vi "Pack Bits x8 (SubVI).vi"(0 "Input Valid?":bool, 2 "Data In":T1, 5 "Bit Depth":u8) -> (14 "Output Valid?":bool, 16 "Data Out":u8[](array[numeric]), 18 "Pixel Sync":bool, 19 "N Bytes":u8)   [LabVIEW 2015]
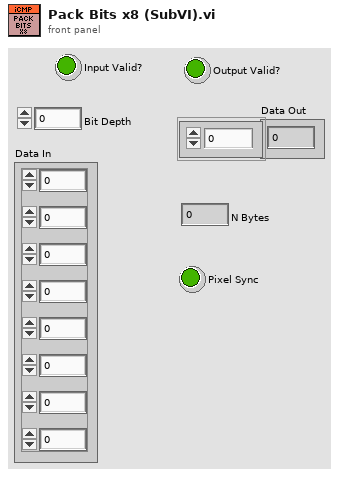
[diagram p1: front panel]
types:
  T1 = cluster{"Numeric Control":u8, "Numeric Control":u8, "Numeric Control":u8, "Numeric Control":u8, "Numeric Control":u8, "Numeric Control":u8, "Numeric Control":u8, "Numeric Control":u8}
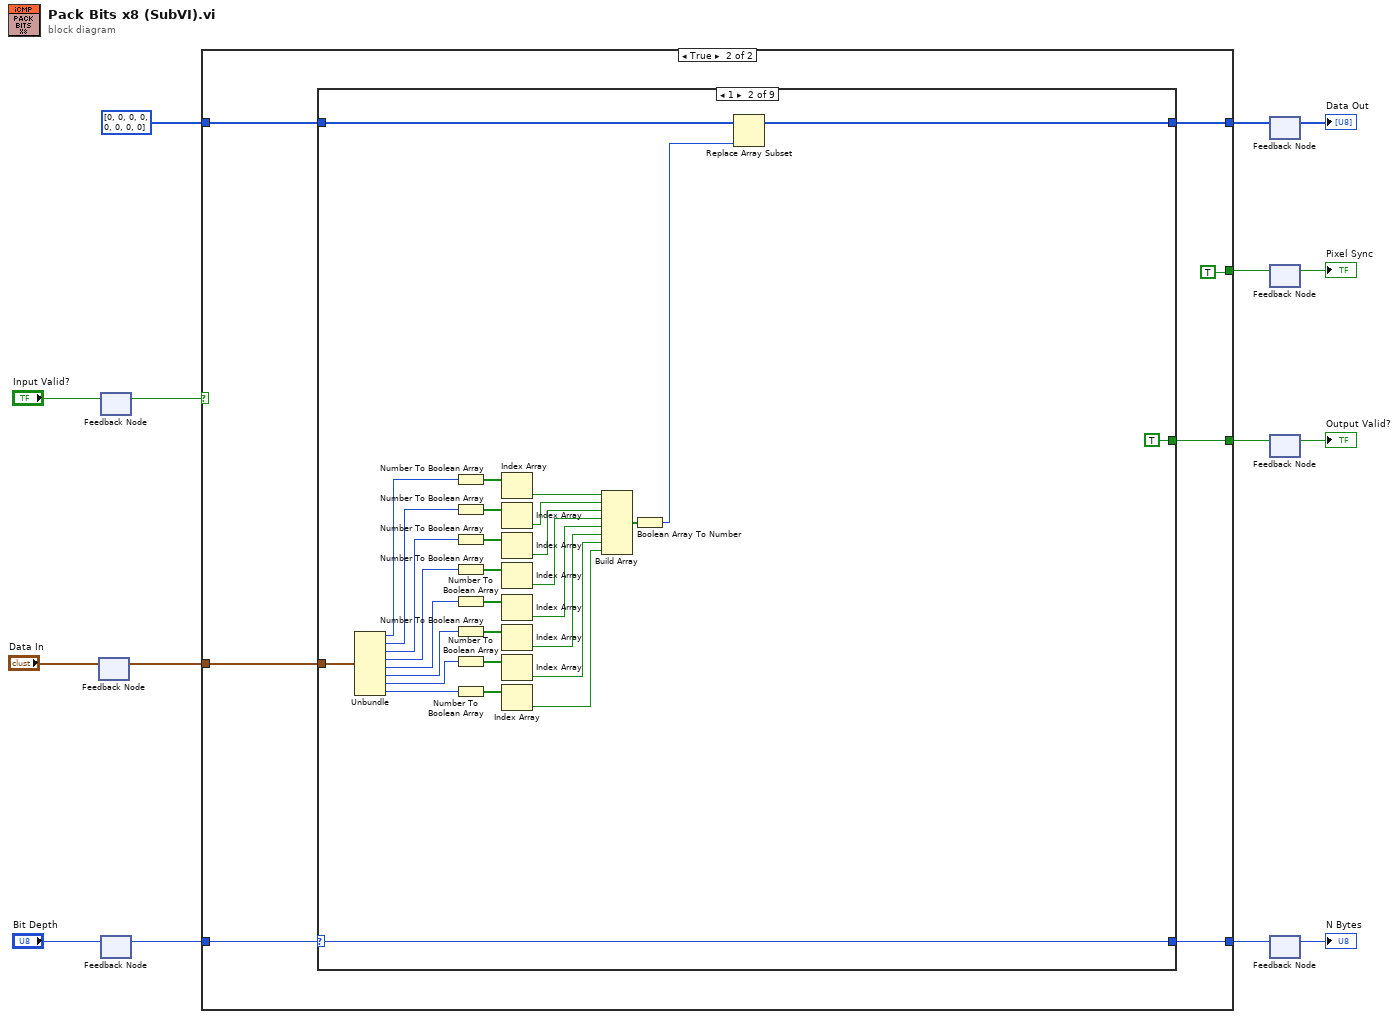
[diagram p0: block diagram]
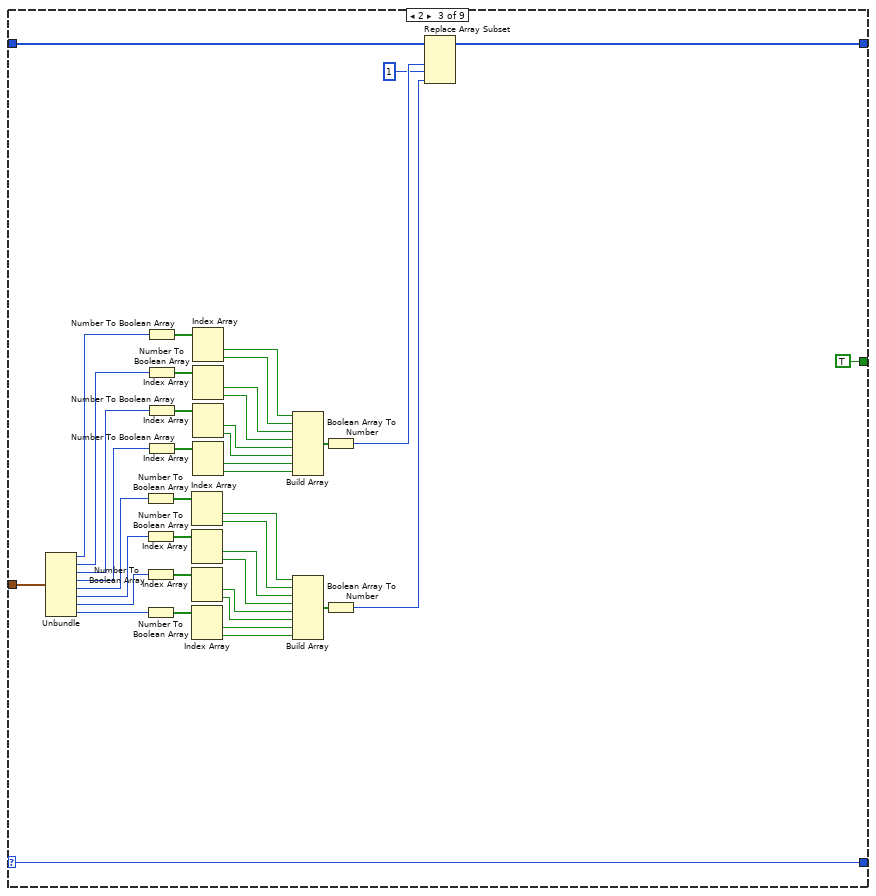
[diagram p4: hidden frame]
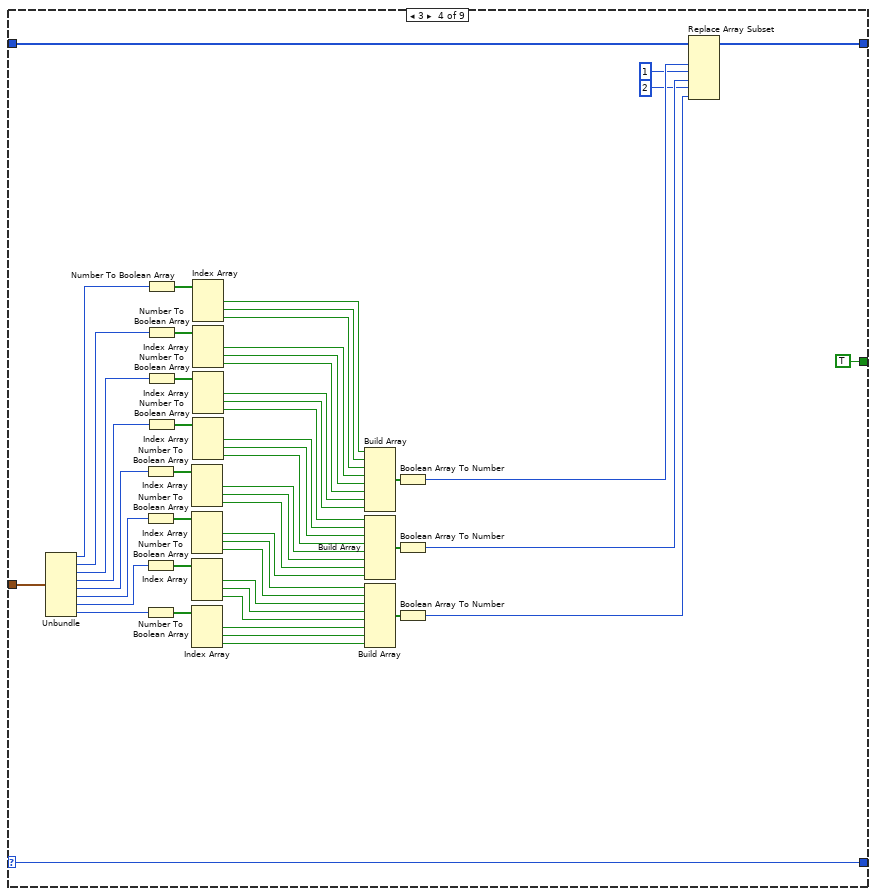
[diagram p5: hidden frame]
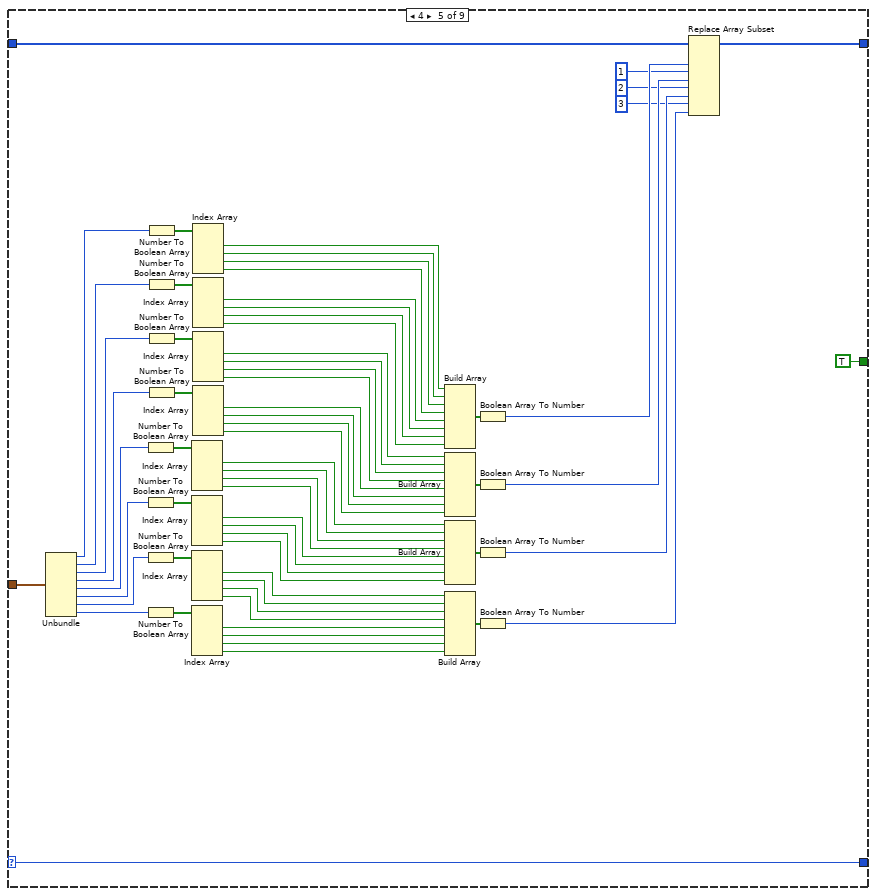
[diagram p6: hidden frame]
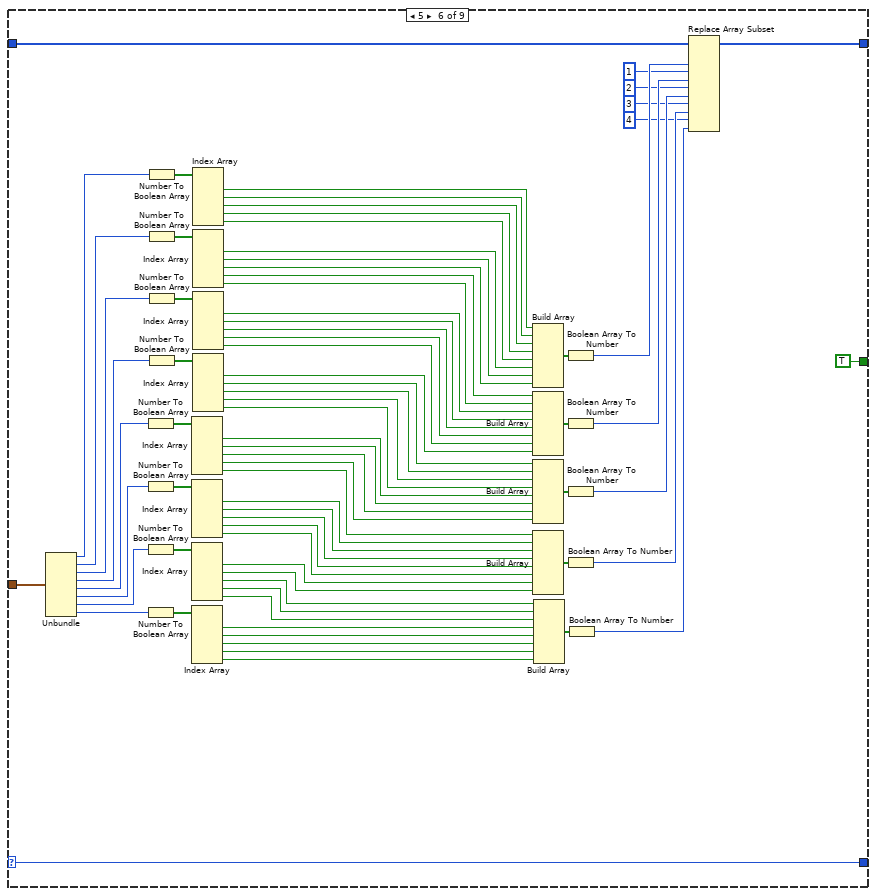
[diagram p7: hidden frame]
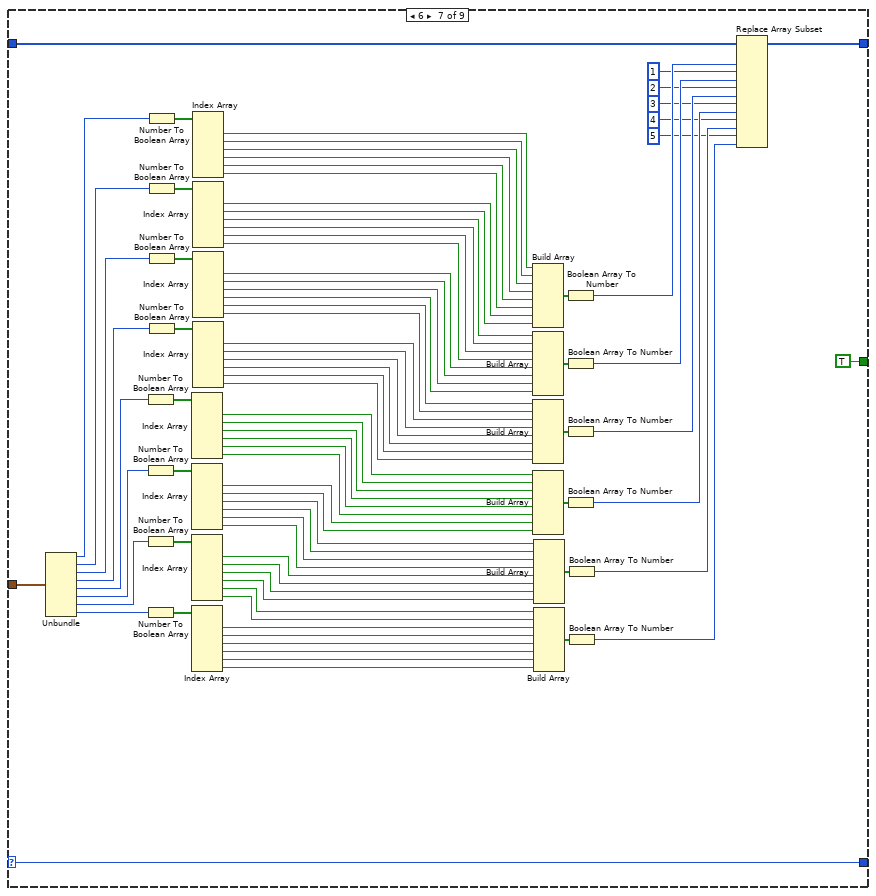
[diagram p8: hidden frame]
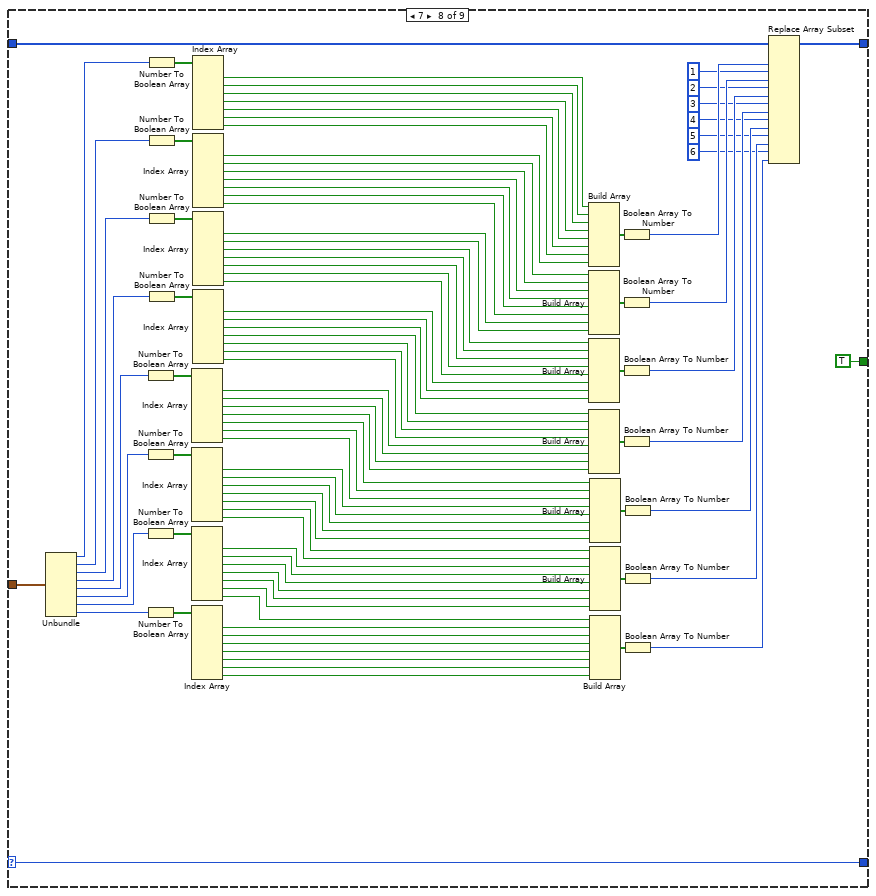
[diagram p9: hidden frame]
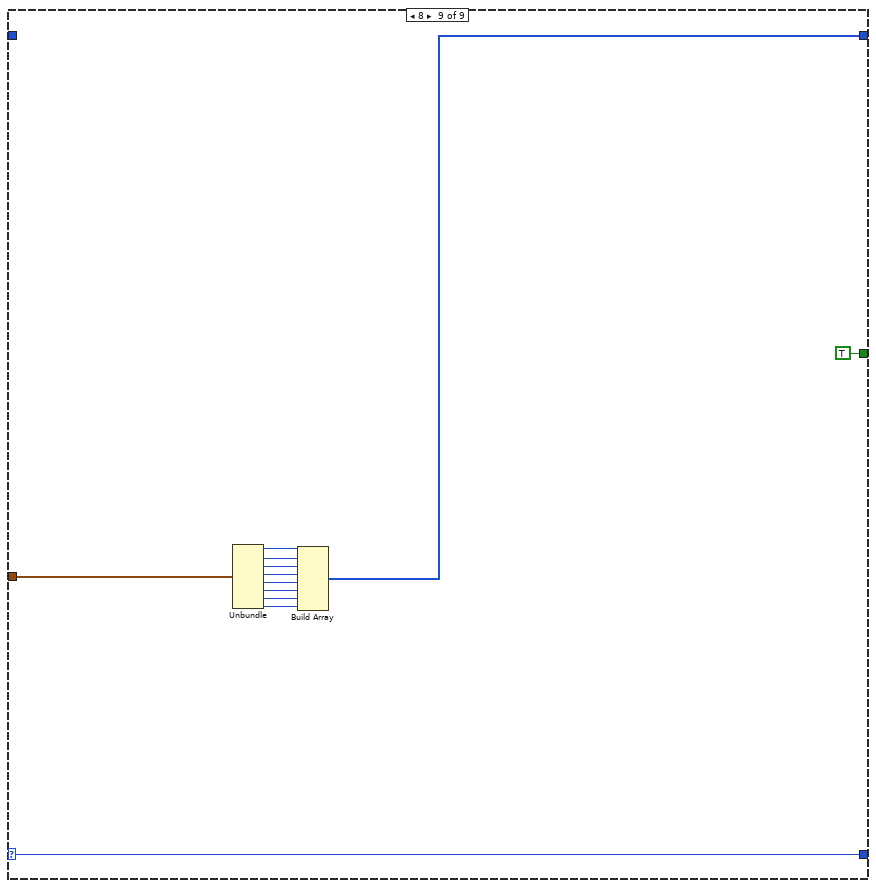
[diagram p10: hidden frame]
diagram:
  n1 = feedback-in #1("Data In") -> ()
  n2 = feedback #1() -> (w11:T1)  [unwired: 1 in]
  n3 = feedback-in #2("Input Valid?") -> ()
  n4 = feedback #2() -> (w13:bool)  [unwired: 1 in]
  n5 = feedback-in #3("Bit Depth") -> ()
  n6 = feedback #3() -> (w10:u8)  [unwired: 1 in]
  n7 = case shown="True" w13 {
    tunnel: [_ w20] -> w8
    tunnel: w11 -> [_ w18]
    tunnel: w10 -> [_ w23]
    tunnel: u8[] [0, 0, 0, 0, 0, 0, 0, 0] -> [w16 w22]
    tunnel: [w16 w21] -> w6
    tunnel: [_ w19] -> w7
    tunnel: [_ TRUE] -> w1
    frame False {
    }
    frame True {
      n8 = case shown="1" w23 {
        selector: w23 -> [w25 w27 w58 w129 w193 w268 w354 w451 w485]
        tunnel: w18 -> [_ w56 w98 w151 w215 w290 w376 w473 w476]
        tunnel: w22 -> [w24 w30 w88 w142 w206 w281 w367 w464 _]
        tunnel: [w24 w28 w86 w140 w204 w279 w365 w462 w475] -> w21
        tunnel: [_ TRUE TRUE TRUE TRUE TRUE TRUE TRUE TRUE] -> w20
        tunnel: [w25 w27 w58 w129 w193 w268 w354 w451 w485] -> w19
        frame 0, Default {
        }
        frame 1 {
          n9 = Unbundle(w56) -> ("Numeric Control"=w55:u8, "Numeric Control"=w52:u8, "Numeric Control"=w49:u8, "Numeric Control"=w48:u8, "Numeric Control"=w43:u8, "Numeric Control"=w42:u8, "Numeric Control"=w41:u8, "Numeric Control"=w40:u8)
          n10 = Number To Boolean Array(number=w55) -> (Boolean array=w54:bool[])
          n11 = Number To Boolean Array(number=w52) -> (Boolean array=w53:bool[])
          n12 = Number To Boolean Array(number=w49) -> (Boolean array=w50:bool[])
          n13 = Number To Boolean Array(number=w48) -> (Boolean array=w51:bool[])
          n14 = Number To Boolean Array(number=w43) -> (Boolean array=w44:bool[])
          n15 = Number To Boolean Array(number=w42) -> (Boolean array=w45:bool[])
          n16 = Number To Boolean Array(number=w41) -> (Boolean array=w47:bool[])
          n17 = Number To Boolean Array(number=w40) -> (Boolean array=w46:bool[])
          n18 = Index Array(array=w54) -> (element=w39:bool)  [unwired: 1 in]
          n19 = Index Array(array=w53) -> (element=w38:bool)  [unwired: 1 in]
          n20 = Index Array(array=w50) -> (element=w37:bool)  [unwired: 1 in]
          n21 = Index Array(array=w51) -> (element=w36:bool)  [unwired: 1 in]
          n22 = Index Array(array=w44) -> (element=w35:bool)  [unwired: 1 in]
          n23 = Index Array(array=w45) -> (element=w34:bool)  [unwired: 1 in]
          n24 = Index Array(array=w47) -> (element=w33:bool)  [unwired: 1 in]
          n25 = Index Array(array=w46) -> (element=w32:bool)  [unwired: 1 in]
          n26 = Build Array(w39, w38, w37, w36, w35, w34, w33, w32) -> (w31:bool[])
          n27 = Boolean Array To Number(Boolean array=w31) -> (number=w29:u8)
          n28 = Replace Array Subset(array=w30, new element=w29) -> (w28:u8[])  [unwired: 1 in]
        }
        frame 2 {
          n29 = Unbundle(w98) -> ("Numeric Control"=w97:u8, "Numeric Control"=w94:u8, "Numeric Control"=w91:u8, "Numeric Control"=w90:u8, "Numeric Control"=w62:u8, "Numeric Control"=w61:u8, "Numeric Control"=w60:u8, "Numeric Control"=w59:u8)
          n30 = Number To Boolean Array(number=w62) -> (Boolean array=w64:bool[])
          n31 = Number To Boolean Array(number=w61) -> (Boolean array=w65:bool[])
          n32 = Number To Boolean Array(number=w60) -> (Boolean array=w67:bool[])
          n33 = Number To Boolean Array(number=w59) -> (Boolean array=w66:bool[])
          n34 = Number To Boolean Array(number=w97) -> (Boolean array=w96:bool[])
          n35 = Number To Boolean Array(number=w94) -> (Boolean array=w95:bool[])
          n36 = Number To Boolean Array(number=w91) -> (Boolean array=w92:bool[])
          n37 = Number To Boolean Array(number=w90) -> (Boolean array=w93:bool[])
          n38 = Index Array(array=w64) -> (element #1=w69:bool, element #2=w70:bool)  [unwired: 2 in]
          n39 = Index Array(array=w65) -> (element #1=w71:bool, element #2=w72:bool)  [unwired: 2 in]
          n40 = Index Array(array=w67) -> (element #1=w73:bool, element #2=w74:bool)  [unwired: 2 in]
          n41 = Index Array(array=w66) -> (element #1=w75:bool, element #2=w76:bool)  [unwired: 2 in]
          n42 = Index Array(array=w96) -> (element #1=w84:bool, element #2=w83:bool)  [unwired: 2 in]
          n43 = Index Array(array=w95) -> (element #1=w82:bool, element #2=w81:bool)  [unwired: 2 in]
          n44 = Index Array(array=w92) -> (element #1=w80:bool, element #2=w79:bool)  [unwired: 2 in]
          n45 = Index Array(array=w93) -> (element #1=w78:bool, element #2=w77:bool)  [unwired: 2 in]
          n46 = Build Array(w84, w83, w82, w81, w80, w79, w78, w77) -> (w89:bool[])
          n47 = Build Array(w69, w70, w71, w72, w73, w74, w75, w76) -> (w68:bool[])
          n48 = Boolean Array To Number(Boolean array=w89) -> (number=w87:u8)
          n49 = Boolean Array To Number(Boolean array=w68) -> (number=w63:u8)
          n50 = Replace Array Subset(array=w88, new element #1=w87, new element #2=w63, index #2=1 ("index")) -> (w86:u8[])  [unwired: 1 in]
        }
        frame 3 {
          n51 = Unbundle(w151) -> ("Numeric Control"=w150:u8, "Numeric Control"=w147:u8, "Numeric Control"=w144:u8, "Numeric Control"=w143:u8, "Numeric Control"=w133:u8, "Numeric Control"=w132:u8, "Numeric Control"=w131:u8, "Numeric Control"=w130:u8)
          n52 = Number To Boolean Array(number=w133) -> (Boolean array=w135:bool[])
          n53 = Number To Boolean Array(number=w132) -> (Boolean array=w136:bool[])
          n54 = Number To Boolean Array(number=w131) -> (Boolean array=w138:bool[])
          n55 = Number To Boolean Array(number=w130) -> (Boolean array=w137:bool[])
          n56 = Number To Boolean Array(number=w150) -> (Boolean array=w149:bool[])
          n57 = Number To Boolean Array(number=w147) -> (Boolean array=w148:bool[])
          n58 = Number To Boolean Array(number=w144) -> (Boolean array=w145:bool[])
          n59 = Number To Boolean Array(number=w143) -> (Boolean array=w146:bool[])
          n60 = Index Array(array=w135) -> (element #1=w114:bool, element #2=w113:bool, element #3=w112:bool)  [unwired: 3 in]
          n61 = Index Array(array=w136) -> (element #1=w111:bool, element #2=w107:bool, element #3=w106:bool)  [unwired: 3 in]
          n62 = Index Array(array=w138) -> (element #1=w105:bool, element #2=w104:bool, element #3=w103:bool)  [unwired: 3 in]
          n63 = Index Array(array=w137) -> (element #1=w102:bool, element #2=w101:bool, element #3=w100:bool)  [unwired: 3 in]
          n64 = Index Array(array=w149) -> (element #1=w126:bool, element #2=w125:bool, element #3=w124:bool)  [unwired: 3 in]
          n65 = Index Array(array=w148) -> (element #1=w123:bool, element #2=w122:bool, element #3=w121:bool)  [unwired: 3 in]
          n66 = Index Array(array=w145) -> (element #1=w120:bool, element #2=w119:bool, element #3=w118:bool)  [unwired: 3 in]
          n67 = Index Array(array=w146) -> (element #1=w117:bool, element #2=w116:bool, element #3=w115:bool)  [unwired: 3 in]
          n68 = Build Array(w126, w125, w124, w123, w122, w121, w120, w119) -> (w128:bool[])
          n69 = Build Array(w118, w117, w116, w115, w114, w113, w112, w111) -> (w127:bool[])
          n70 = Build Array(w107, w106, w105, w104, w103, w102, w101, w100) -> (w109:bool[])
          n71 = Boolean Array To Number(Boolean array=w128) -> (number=w141:u8)
          n72 = Boolean Array To Number(Boolean array=w127) -> (number=w134:u8)
          n73 = Boolean Array To Number(Boolean array=w109) -> (number=w108:u8)
          n74 = Replace Array Subset(array=w142, new element #1=w141, new element #2=w134, index #2=1 ("index"), new element #3=w108, index #3=2 ("index")) -> (w140:u8[])  [unwired: 1 in]
        }
        frame 4 {
          n75 = Unbundle(w215) -> ("Numeric Control"=w214:u8, "Numeric Control"=w211:u8, "Numeric Control"=w208:u8, "Numeric Control"=w207:u8, "Numeric Control"=w197:u8, "Numeric Control"=w196:u8, "Numeric Control"=w195:u8, "Numeric Control"=w194:u8)
          n76 = Number To Boolean Array(number=w197) -> (Boolean array=w199:bool[])
          n77 = Number To Boolean Array(number=w196) -> (Boolean array=w200:bool[])
          n78 = Number To Boolean Array(number=w195) -> (Boolean array=w202:bool[])
          n79 = Number To Boolean Array(number=w194) -> (Boolean array=w201:bool[])
          n80 = Number To Boolean Array(number=w214) -> (Boolean array=w213:bool[])
          n81 = Number To Boolean Array(number=w211) -> (Boolean array=w212:bool[])
          n82 = Number To Boolean Array(number=w208) -> (Boolean array=w209:bool[])
          n83 = Number To Boolean Array(number=w207) -> (Boolean array=w210:bool[])
          n84 = Index Array(array=w199) -> (element #1=w168:bool, element #2=w167:bool, element #3=w166:bool, element #4=w165:bool)  [unwired: 4 in]
          n85 = Index Array(array=w200) -> (element #1=w164:bool, element #2=w163:bool, element #3=w162:bool, element #4=w161:bool)  [unwired: 4 in]
          n86 = Index Array(array=w202) -> (element #1=w160:bool, element #2=w159:bool, element #3=w158:bool, element #4=w157:bool)  [unwired: 4 in]
          n87 = Index Array(array=w201) -> (element #1=w156:bool, element #2=w155:bool, element #3=w154:bool, element #4=w153:bool)  [unwired: 4 in]
          n88 = Index Array(array=w213) -> (element #1=w190:bool, element #2=w189:bool, element #3=w188:bool, element #4=w181:bool)  [unwired: 4 in]
          n89 = Index Array(array=w212) -> (element #1=w180:bool, element #2=w179:bool, element #3=w178:bool, element #4=w177:bool)  [unwired: 4 in]
          n90 = Index Array(array=w209) -> (element #1=w176:bool, element #2=w175:bool, element #3=w174:bool, element #4=w173:bool)  [unwired: 4 in]
          n91 = Index Array(array=w210) -> (element #1=w172:bool, element #2=w171:bool, element #3=w170:bool, element #4=w169:bool)  [unwired: 4 in]
          n92 = Build Array(w190, w189, w188, w181, w180, w179, w178, w177) -> (w192:bool[])
          n93 = Build Array(w176, w175, w174, w173, w172, w171, w170, w169) -> (w191:bool[])
          n94 = Build Array(w168, w167, w166, w165, w164, w163, w162, w161) -> (w186:bool[])
          n95 = Build Array(w160, w159, w158, w157, w156, w155, w154, w153) -> (w184:bool[])
          n96 = Boolean Array To Number(Boolean array=w192) -> (number=w205:u8)
          n97 = Boolean Array To Number(Boolean array=w191) -> (number=w198:u8)
          n98 = Boolean Array To Number(Boolean array=w186) -> (number=w185:u8)
          n99 = Boolean Array To Number(Boolean array=w184) -> (number=w182:u8)
          n100 = Replace Array Subset(array=w206, new element #1=w205, new element #2=w198, index #2=1 ("index"), new element #3=w185, index #3=2 ("index"), new element #4=w182, index #4=3 ("index")) -> (w204:u8[])  [unwired: 1 in]
        }
        frame 5 {
          n101 = Unbundle(w290) -> ("Numeric Control"=w289:u8, "Numeric Control"=w286:u8, "Numeric Control"=w283:u8, "Numeric Control"=w282:u8, "Numeric Control"=w272:u8, "Numeric Control"=w271:u8, "Numeric Control"=w270:u8, "Numeric Control"=w269:u8)
          n102 = Number To Boolean Array(number=w272) -> (Boolean array=w274:bool[])
          n103 = Number To Boolean Array(number=w271) -> (Boolean array=w275:bool[])
          n104 = Number To Boolean Array(number=w270) -> (Boolean array=w277:bool[])
          n105 = Number To Boolean Array(number=w269) -> (Boolean array=w276:bool[])
          n106 = Number To Boolean Array(number=w289) -> (Boolean array=w288:bool[])
          n107 = Number To Boolean Array(number=w286) -> (Boolean array=w287:bool[])
          n108 = Number To Boolean Array(number=w283) -> (Boolean array=w284:bool[])
          n109 = Number To Boolean Array(number=w282) -> (Boolean array=w285:bool[])
          n110 = Index Array(array=w274) -> (element #1=w236:bool, element #2=w235:bool, element #3=w234:bool, element #4=w233:bool, element #5=w232:bool)  [unwired: 5 in]
          n111 = Index Array(array=w275) -> (element #1=w231:bool, element #2=w230:bool, element #3=w229:bool, element #4=w228:bool, element #5=w227:bool)  [unwired: 5 in]
          n112 = Index Array(array=w277) -> (element #1=w226:bool, element #2=w225:bool, element #3=w224:bool, element #4=w223:bool, element #5=w222:bool)  [unwired: 5 in]
          n113 = Index Array(array=w276) -> (element #1=w221:bool, element #2=w220:bool, element #3=w219:bool, element #4=w218:bool, element #5=w217:bool)  [unwired: 5 in]
          n114 = Index Array(array=w288) -> (element #1=w265:bool, element #2=w264:bool, element #3=w263:bool, element #4=w256:bool, element #5=w252:bool)  [unwired: 5 in]
          n115 = Index Array(array=w287) -> (element #1=w251:bool, element #2=w250:bool, element #3=w249:bool, element #4=w248:bool, element #5=w247:bool)  [unwired: 5 in]
          n116 = Index Array(array=w284) -> (element #1=w246:bool, element #2=w245:bool, element #3=w244:bool, element #4=w243:bool, element #5=w242:bool)  [unwired: 5 in]
          n117 = Index Array(array=w285) -> (element #1=w241:bool, element #2=w240:bool, element #3=w239:bool, element #4=w238:bool, element #5=w237:bool)  [unwired: 5 in]
          n118 = Build Array(w265, w264, w263, w256, w252, w251, w250, w249) -> (w267:bool[])
          n119 = Build Array(w248, w247, w246, w245, w244, w243, w242, w241) -> (w266:bool[])
          n120 = Build Array(w240, w239, w238, w237, w236, w235, w234, w233) -> (w261:bool[])
          n121 = Build Array(w232, w231, w230, w229, w228, w227, w226, w225) -> (w259:bool[])
          n122 = Build Array(w224, w223, w222, w221, w220, w219, w218, w217) -> (w255:bool[])
          n123 = Boolean Array To Number(Boolean array=w267) -> (number=w280:u8)
          n124 = Boolean Array To Number(Boolean array=w266) -> (number=w273:u8)
          n125 = Boolean Array To Number(Boolean array=w261) -> (number=w260:u8)
          n126 = Boolean Array To Number(Boolean array=w259) -> (number=w257:u8)
          n127 = Boolean Array To Number(Boolean array=w255) -> (number=w253:u8)
          n128 = Replace Array Subset(array=w281, new element #1=w280, new element #2=w273, index #2=1 ("index"), new element #3=w260, index #3=2 ("index"), new element #4=w257, index #4=3 ("index"), new element #5=w253, index #5=4 ("index")) -> (w279:u8[])  [unwired: 1 in]
        }
        frame 6 {
          n129 = Unbundle(w376) -> ("Numeric Control"=w375:u8, "Numeric Control"=w372:u8, "Numeric Control"=w369:u8, "Numeric Control"=w368:u8, "Numeric Control"=w358:u8, "Numeric Control"=w357:u8, "Numeric Control"=w356:u8, "Numeric Control"=w355:u8)
          n130 = Number To Boolean Array(number=w358) -> (Boolean array=w360:bool[])
          n131 = Number To Boolean Array(number=w357) -> (Boolean array=w361:bool[])
          n132 = Number To Boolean Array(number=w356) -> (Boolean array=w363:bool[])
          n133 = Number To Boolean Array(number=w355) -> (Boolean array=w362:bool[])
          n134 = Number To Boolean Array(number=w375) -> (Boolean array=w374:bool[])
          n135 = Number To Boolean Array(number=w372) -> (Boolean array=w373:bool[])
          n136 = Number To Boolean Array(number=w369) -> (Boolean array=w370:bool[])
          n137 = Number To Boolean Array(number=w368) -> (Boolean array=w371:bool[])
          n138 = Index Array(array=w360) -> (element #1=w315:bool, element #2=w314:bool, element #3=w313:bool, element #4=w312:bool, element #5=w311:bool, element #6=w310:bool)  [unwired: 6 in]
          n139 = Index Array(array=w361) -> (element #1=w309:bool, element #2=w308:bool, element #3=w307:bool, element #4=w306:bool, element #5=w305:bool, element #6=w304:bool)  [unwired: 6 in]
          n140 = Index Array(array=w363) -> (element #1=w303:bool, element #2=w302:bool, element #3=w301:bool, element #4=w300:bool, element #5=w299:bool, element #6=w298:bool)  [unwired: 6 in]
          n141 = Index Array(array=w362) -> (element #1=w297:bool, element #2=w296:bool, element #3=w295:bool, element #4=w294:bool, element #5=w293:bool, element #6=w292:bool)  [unwired: 6 in]
          n142 = Index Array(array=w374) -> (element #1=w351:bool, element #2=w350:bool, element #3=w349:bool, element #4=w342:bool, element #5=w338:bool, element #6=w334:bool)  [unwired: 6 in]
          n143 = Index Array(array=w373) -> (element #1=w333:bool, element #2=w332:bool, element #3=w331:bool, element #4=w330:bool, element #5=w329:bool, element #6=w328:bool)  [unwired: 6 in]
          n144 = Index Array(array=w370) -> (element #1=w327:bool, element #2=w326:bool, element #3=w325:bool, element #4=w324:bool, element #5=w323:bool, element #6=w322:bool)  [unwired: 6 in]
          n145 = Index Array(array=w371) -> (element #1=w321:bool, element #2=w320:bool, element #3=w319:bool, element #4=w318:bool, element #5=w317:bool, element #6=w316:bool)  [unwired: 6 in]
          n146 = Build Array(w351, w350, w349, w342, w338, w334, w333, w332) -> (w353:bool[])
          n147 = Build Array(w331, w330, w329, w328, w327, w326, w325, w324) -> (w352:bool[])
          n148 = Build Array(w323, w322, w321, w320, w319, w318, w317, w316) -> (w347:bool[])
          n149 = Build Array(w315, w314, w313, w312, w311, w310, w309, w308) -> (w345:bool[])
          n150 = Build Array(w307, w306, w305, w304, w303, w302, w301, w300) -> (w341:bool[])
          n151 = Build Array(w299, w298, w297, w296, w295, w294, w293, w292) -> (w336:bool[])
          n152 = Boolean Array To Number(Boolean array=w353) -> (number=w366:u8)
          n153 = Boolean Array To Number(Boolean array=w352) -> (number=w359:u8)
          n154 = Boolean Array To Number(Boolean array=w347) -> (number=w346:u8)
          n155 = Boolean Array To Number(Boolean array=w345) -> (number=w343:u8)
          n156 = Boolean Array To Number(Boolean array=w341) -> (number=w339:u8)
          n157 = Boolean Array To Number(Boolean array=w336) -> (number=w335:u8)
          n158 = Replace Array Subset(array=w367, new element #1=w366, new element #2=w359, index #2=1 ("index"), new element #3=w346, index #3=2 ("index"), new element #4=w343, index #4=3 ("index"), new element #5=w339, index #5=4 ("index"), new element #6=w335, index #6=5 ("index")) -> (w365:u8[])  [unwired: 1 in]
        }
        frame 7 {
          n159 = Unbundle(w473) -> ("Numeric Control"=w472:u8, "Numeric Control"=w469:u8, "Numeric Control"=w466:u8, "Numeric Control"=w465:u8, "Numeric Control"=w455:u8, "Numeric Control"=w454:u8, "Numeric Control"=w453:u8, "Numeric Control"=w452:u8)
          n160 = Number To Boolean Array(number=w455) -> (Boolean array=w457:bool[])
          n161 = Number To Boolean Array(number=w454) -> (Boolean array=w458:bool[])
          n162 = Number To Boolean Array(number=w453) -> (Boolean array=w460:bool[])
          n163 = Number To Boolean Array(number=w452) -> (Boolean array=w459:bool[])
          n164 = Number To Boolean Array(number=w472) -> (Boolean array=w471:bool[])
          n165 = Number To Boolean Array(number=w469) -> (Boolean array=w470:bool[])
          n166 = Number To Boolean Array(number=w466) -> (Boolean array=w467:bool[])
          n167 = Number To Boolean Array(number=w465) -> (Boolean array=w468:bool[])
          n168 = Index Array(array=w457) -> (element #1=w405:bool, element #2=w404:bool, element #3=w403:bool, element #4=w402:bool, element #5=w401:bool, element #6=w400:bool, element #7=w399:bool)  [unwired: 7 in]
          n169 = Index Array(array=w458) -> (element #1=w398:bool, element #2=w397:bool, element #3=w396:bool, element #4=w395:bool, element #5=w394:bool, element #6=w393:bool, element #7=w392:bool)  [unwired: 7 in]
          n170 = Index Array(array=w460) -> (element #1=w391:bool, element #2=w390:bool, element #3=w389:bool, element #4=w388:bool, element #5=w387:bool, element #6=w386:bool, element #7=w385:bool)  [unwired: 7 in]
          n171 = Index Array(array=w459) -> (element #1=w384:bool, element #2=w383:bool, element #3=w382:bool, element #4=w381:bool, element #5=w380:bool, element #6=w379:bool, element #7=w378:bool)  [unwired: 7 in]
          n172 = Index Array(array=w471) -> (element #1=w448:bool, element #2=w447:bool, element #3=w446:bool, element #4=w439:bool, element #5=w435:bool, element #6=w431:bool, element #7=w427:bool)  [unwired: 7 in]
          n173 = Index Array(array=w470) -> (element #1=w426:bool, element #2=w425:bool, element #3=w424:bool, element #4=w423:bool, element #5=w422:bool, element #6=w421:bool, element #7=w420:bool)  [unwired: 7 in]
          n174 = Index Array(array=w467) -> (element #1=w419:bool, element #2=w418:bool, element #3=w417:bool, element #4=w416:bool, element #5=w415:bool, element #6=w414:bool, element #7=w413:bool)  [unwired: 7 in]
          n175 = Index Array(array=w468) -> (element #1=w412:bool, element #2=w411:bool, element #3=w410:bool, element #4=w409:bool, element #5=w408:bool, element #6=w407:bool, element #7=w406:bool)  [unwired: 7 in]
          n176 = Build Array(w448, w447, w446, w439, w435, w431, w427, w426) -> (w450:bool[])
          n177 = Build Array(w425, w424, w423, w422, w421, w420, w419, w418) -> (w449:bool[])
          n178 = Build Array(w417, w416, w415, w414, w413, w412, w411, w410) -> (w444:bool[])
          n179 = Build Array(w409, w408, w407, w406, w405, w404, w403, w402) -> (w442:bool[])
          n180 = Build Array(w401, w400, w399, w398, w397, w396, w395, w394) -> (w438:bool[])
          n181 = Build Array(w393, w392, w391, w390, w389, w388, w387, w386) -> (w433:bool[])
          n182 = Build Array(w385, w384, w383, w382, w381, w380, w379, w378) -> (w429:bool[])
          n183 = Boolean Array To Number(Boolean array=w450) -> (number=w463:u8)
          n184 = Boolean Array To Number(Boolean array=w449) -> (number=w456:u8)
          n185 = Boolean Array To Number(Boolean array=w444) -> (number=w443:u8)
          n186 = Boolean Array To Number(Boolean array=w442) -> (number=w440:u8)
          n187 = Boolean Array To Number(Boolean array=w438) -> (number=w436:u8)
          n188 = Boolean Array To Number(Boolean array=w433) -> (number=w432:u8)
          n189 = Boolean Array To Number(Boolean array=w429) -> (number=w428:u8)
          n190 = Replace Array Subset(array=w464, new element #1=w463, new element #2=w456, index #2=1 ("index"), new element #3=w443, index #3=2 ("index"), new element #4=w440, index #4=3 ("index"), new element #5=w436, index #5=4 ("index"), new element #6=w432, index #6=5 ("index"), new element #7=w428, index #7=6 ("index")) -> (w462:u8[])  [unwired: 1 in]
        }
        frame 8 {
          n191 = Unbundle(w476) -> ("Numeric Control"=w484:u8, "Numeric Control"=w483:u8, "Numeric Control"=w482:u8, "Numeric Control"=w481:u8, "Numeric Control"=w480:u8, "Numeric Control"=w479:u8, "Numeric Control"=w478:u8, "Numeric Control"=w477:u8)
          n192 = Build Array(w484, w483, w482, w481, w480, w479, w478, w477) -> (w475:u8[])
        }
      }
    }
  }
  n193 = feedback-in #4(w6) -> ()
  n194 = feedback #4() -> (→"Data Out":u8[])  [unwired: 1 in]
  n195 = feedback #5() -> (→"Pixel Sync":bool)  [unwired: 1 in]
  n196 = feedback-in #5(w1) -> ()
  n197 = feedback-in #6(w8) -> ()
  n198 = feedback #6() -> (→"Output Valid?":bool)  [unwired: 1 in]
  n199 = feedback-in #7(w7) -> ()
  n200 = feedback #7() -> (→"N Bytes":u8)  [unwired: 1 in]
